vi "Manual Assembly DB new.vi"() -> ()   [LabVIEW 2021]
uses:
  Classes/Routine/Routine Enum.ctl
  Classes/Assembly/Database Entry/Database Entry.lvclass
  Classes/Assembly/Assembly Run.lvclass
  Classes/Workspace/Fixture Enum.ctl
  <vilib>/Utility/file.llb/Read Delimited Spreadsheet (string).vi
  SubVIs/PUT_region.vi
  SubVIs/component_tray_region.vi
  SubVIs/assembly_tray_region.vi
  Classes/Routine/Routine.lvclass
  Classes/Workspace/Fixture.lvclass
  Classes/Controller/Controller.lvclass
  <vilib>/JDP Science/JDP Science Common Utilities/JDP Utility.lvlib
panel:
  out "Stack names":T1
  out "Feet check":bool
  out "Assembly Type":string[](array[string])
  out "Assembly tray region":dbl
  out "Component tray region":dbl
  out "PUT Region":dbl
  in  "Clear All":bool
  in  "Assemble":bool
  in  "Pick and Place":bool
  in  "Dispense glue":bool
  in  "Go":bool
  in  "Routine":T2=enum."Dispense Epoxy"
  in  "Update":bool
  in  "Stage":i32(listbox)=-1
  in  "Stop":bool
  in  "Remove":bool
  in  "Add":bool
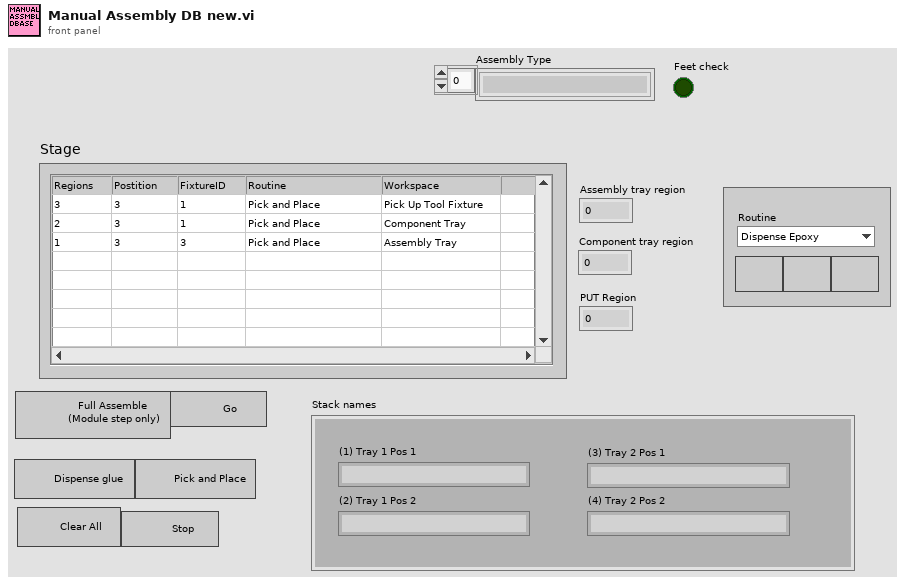
[diagram p1: front panel]
types:
  T1 = cluster{"(1) Tray 1 Pos 1":string, "(2) Tray 1 Pos 2":string, "(3) Tray 2 Pos 1":string, "(4) Tray 2 Pos 2":string}
  T2 = typedef "Routine.lvclass/Routine Enum.ctl" = enum16{"Primary Pick Up", "Secondary Pick Up", "Put Down All", "Secure Syringe", "Release Syringe", "Dispense Epoxy", "Pick Up All", "Put Down Secondary", "Full Assembly"}
  T3 = typedef "Fixture.lvclass/Fixture Enum.ctl" = enum16{"Assembly Tray", "Syringe Space", "Component", "Pick Up Tool", "Current Position"}
  T4 = typedef "File Paths.ctl" = cluster{"Glue Pattern Folder":path, "Carrier Tray Folder":path, "Pick Up Tool Fixture Folder":path, "Components Folder":path, "Bellows Tool Offset.txt":path, "Pick Up Tool Offset.txt":path, "Dispense Tip Offset.txt":path, "Log Files":path, "Gantry Assembly Map.txt":path, "Syringe and offset map.txt":path, "Controllers Folder":path, "Local dbase config":path}
  T5 = cluster{"Fixture ID":dbl, "Position":dbl, "Thickness":dbl}[]
  T6 = cluster{"Stack names[0]":string, "Stack names[1]":string, "Stack names[2]":string, "Stack names[3]":string}
  T7 = typedef "Controller.lvclass/Controllers.ctl" = cluster{"I-O.lvclass":refnum<class "I-O.lvclass">, "Gantry":refnum<k24>, "Dispenser":refnum<visa-resource-name>}
  T8 = cluster{"Fixture ID":dbl, "Position":dbl, "Thickness":dbl}
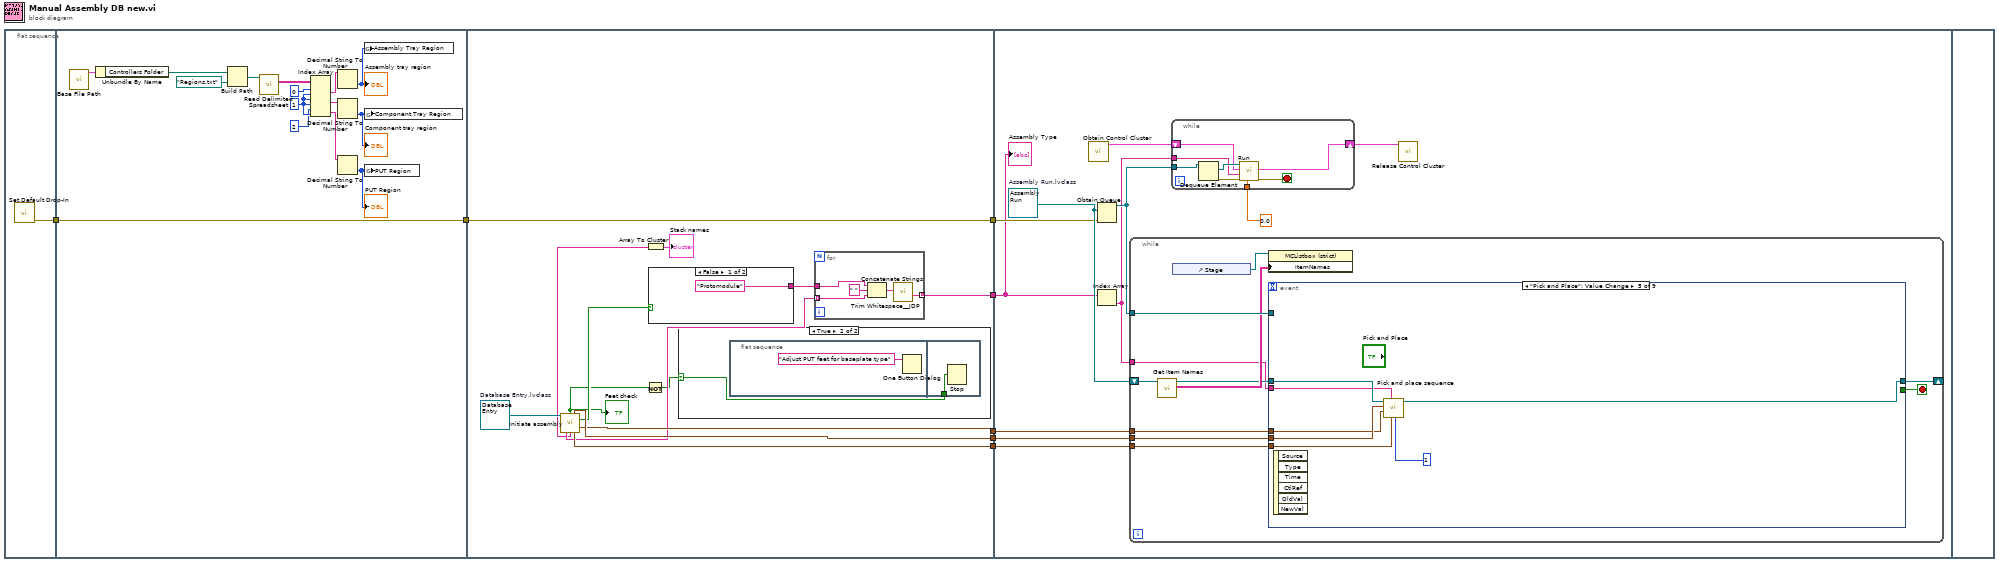
[diagram p0: block diagram]
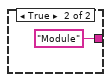
[diagram p3: hidden frame]
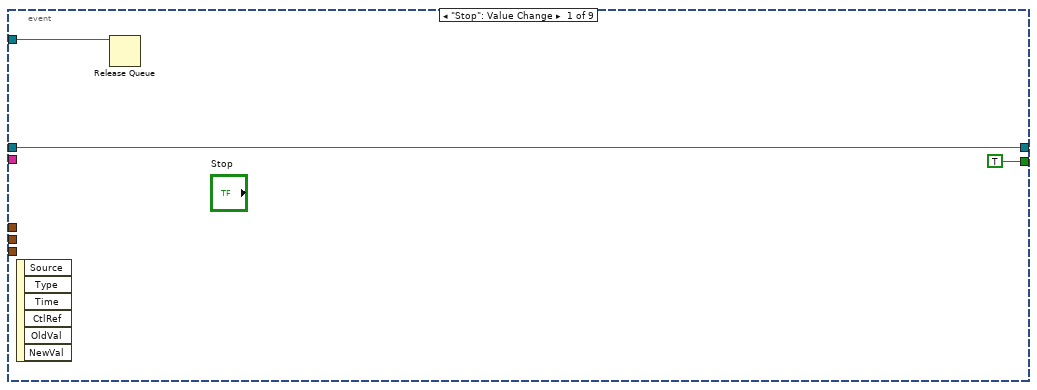
[diagram p4: hidden frame]
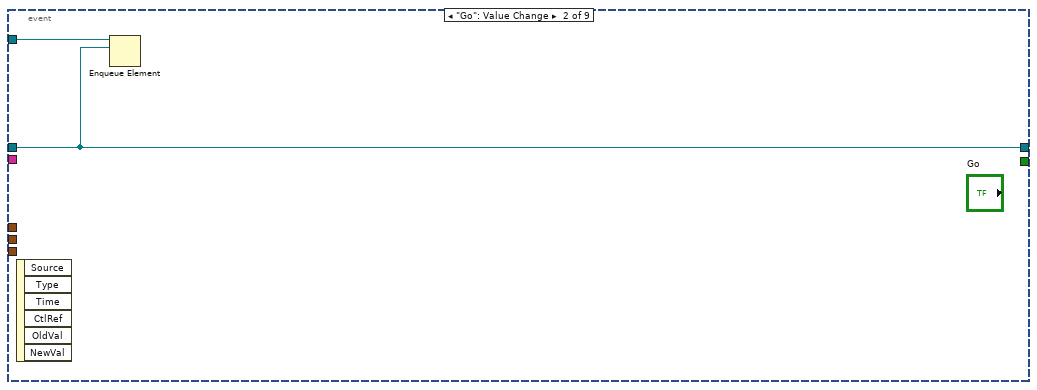
[diagram p5: hidden frame]
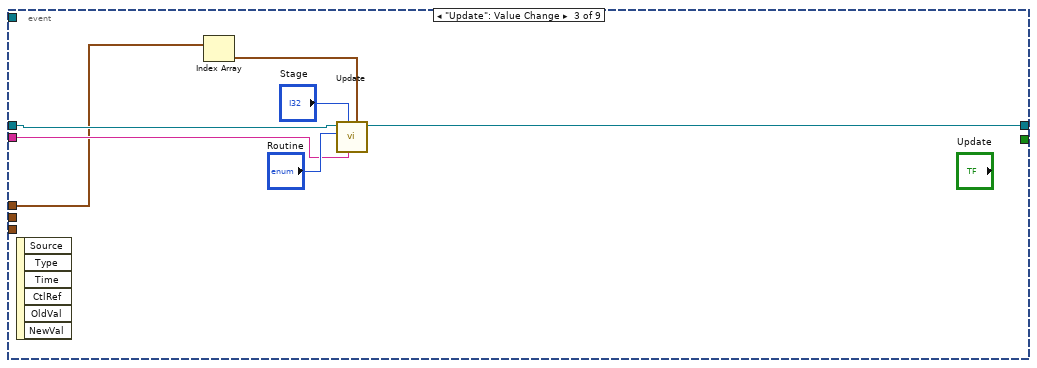
[diagram p6: hidden frame]
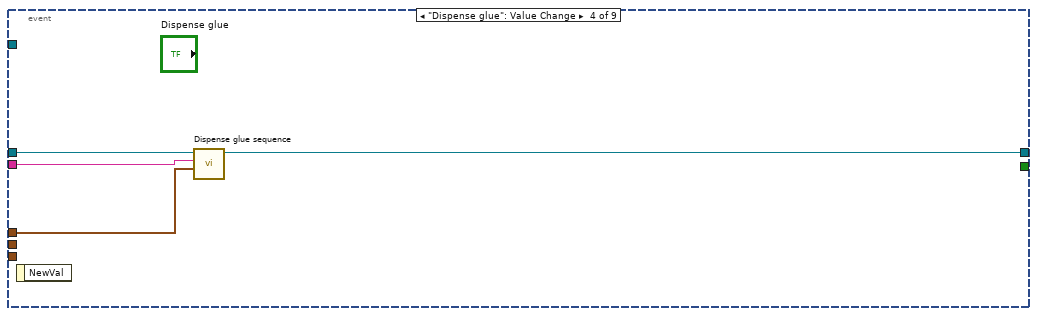
[diagram p7: hidden frame]
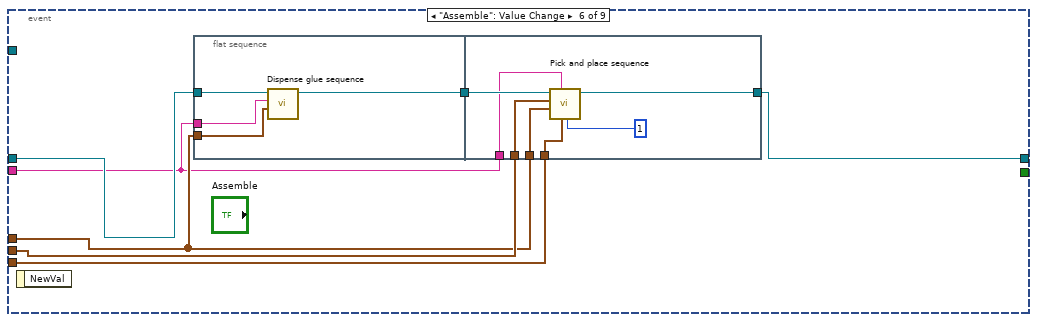
[diagram p8: hidden frame]
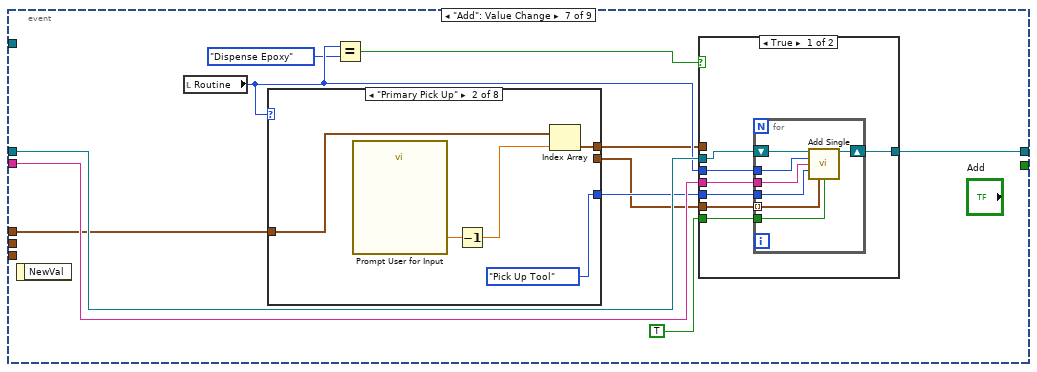
[diagram p9: hidden frame]
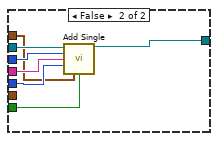
[diagram p10: hidden frame]
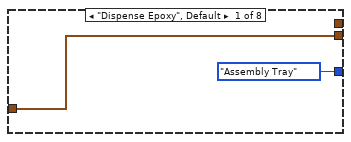
[diagram p11: hidden frame]
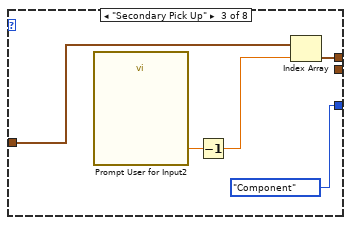
[diagram p12: hidden frame]
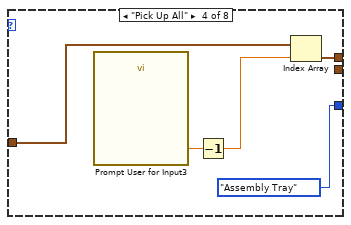
[diagram p13: hidden frame]
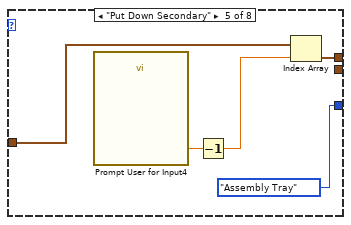
[diagram p14: hidden frame]
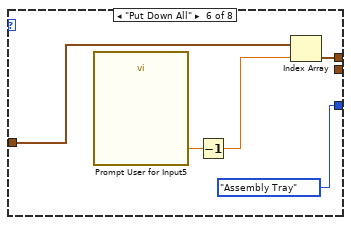
[diagram p15: hidden frame]
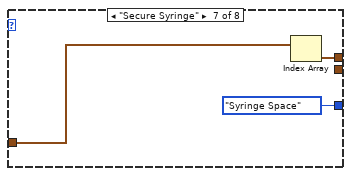
[diagram p16: hidden frame]
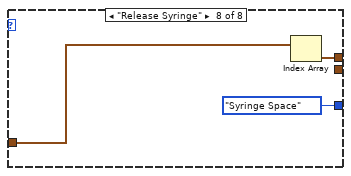
[diagram p17: hidden frame]
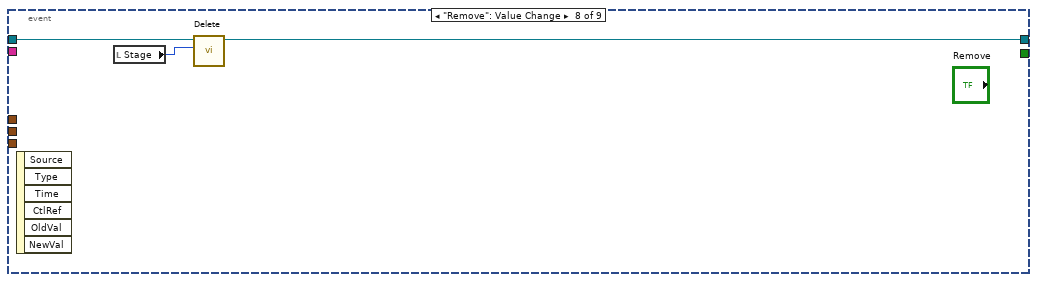
[diagram p18: hidden frame]
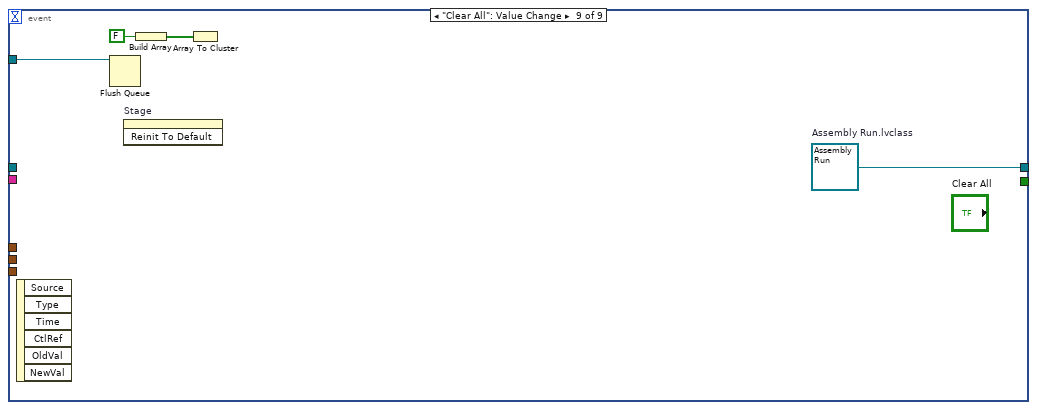
[diagram p19: hidden frame]
diagram:
  n1 = flat-sequence {
    tunnel: [w8] -> w5
    tunnel: [w9] -> w6
    tunnel: w5 -> [w9]
    tunnel: [w35] -> w7
    tunnel: w6 -> [w35]
    tunnel: [w34] -> w4
    tunnel: [w33] -> w3
    tunnel: [w32] -> w2
    tunnel: [w28] -> w1
    tunnel: w7 -> [w53]
    tunnel: w4 -> [w52]
    tunnel: w3 -> [w51]
    tunnel: w2 -> [w50]
    tunnel: w1 -> [w49]
    frame #0 {
      n2 = call "Set Default Drop-In.vi"() -> ("error out"=w8:errorcluster)  [unwired: 11 in]
    }
    frame #1 {
      w12 = 1 ("disabled index (col)")
      n3 = call "Base File Path.vi"() -> ("Paths Out"=w23:T4)  [unwired: 11 in]
      n4 = Unbundle By Name(w23) -> ("Controllers Folder"=w21:path)
      n5 = Build Path(base path=w21, name or relative path=path "Regions.txt") -> (appended path=w22:path)
      n6 = call-poly <vilib>:"Read Delimited Spreadsheet.vi"("file path (dialog if empty)"=w22) -> ("all rows"=w10:string[][])  [unwired: 9 in, 5 out]
      n7 = Index Array(array=w10, index (row) #1=0 ("index (row)"), index (col) #1=w12, index (row) #2=w12, index (col) #2=w12, index (row) #3=2 ("disabled index (row)"), index (col) #3=w12) -> (element #1=w15:string, element #2=w14:string, element #3=w16:string)
      n8 = Decimal String To Number(string=w15) -> (number=w18:i32)  [unwired: 2 in, 1 out]
      "Assembly tray region" <- w18
      n9 = Decimal String To Number(string=w14) -> (number=w19:i32)  [unwired: 2 in, 1 out]
      "Component tray region" <- w19
      n10 = Decimal String To Number(string=w16) -> (number=w17:i32)  [unwired: 2 in, 1 out]
      "PUT Region" <- w17
      n11 = global write "assembly_tray_region.vi" "Assembly Tray Region"(w18) -> ()
      n12 = global write "component_tray_region.vi" "Component Tray Region"(w19) -> ()
      n13 = global write "PUT_region.vi" "PUT Region"(w17) -> ()
    }
    frame #2 {
      w36 = refnum<class "Database Entry.lvclass"> refnum  # Database Entry.lvclass
      n14 = call "Initiate assembly.vi"("Database Entry in"=w36) -> ("Feet check"=w24:bool, "PUT Settings"=w33:T5, "Module?"=w31:bool, "Assembly Settings"=w32:T5, "Assembly Type"=w30:string[], "Stack names"=w25:string[], "Component Settings"=w34:T5)  [unwired: 5 in, 3 out]
      "Feet check" <- w24
      n15 = Array To Cluster(array=w25) -> (cluster=→"Stack names":T6)
      n16 = Not(x=w24) -> (.not. x?=w27:bool)
      n17 = case shown="False" w31 {
        tunnel: ["Protomodule" "Module"] -> w29
        frame False {
        }
        frame True {
        }
      }
      n18 = case shown="True" w27 {
        selector: w27 -> [_ w37]
        frame False {
        }
        frame True {
          n19 = flat-sequence {
            tunnel: w37 -> [w39]
            frame #0 {
              n20 = One Button Dialog(message="Adjust PUT feet for baseplate type") -> ()  [unwired: 1 in, 1 out]
            }
            frame #1 {
              n21 = Stop(stop? (T)=w39) -> ()
            }
          }
        }
      }
      n22 = for {
        tunnel: w30 -> [w42] mode=indexing
        tunnel: w29 -> [w44]
        tunnel: [w40] -> w28 mode=indexing
        n23 = Concatenate Strings(w44, " " ("string"), w42) -> (w41:string)
        n24 = call <vilib>:"Trim Whitespace__JDP.vi"("String in"=w41) -> ("String out"=w40:string)  [unwired: 6 in]
      }
    }
    frame #3 {
      w55 = refnum<class "Assembly Run.lvclass"> refnum  # Assembly Run.lvclass
      n25 = call "Obtain Control Cluster.vi"() -> ("Control Out"=w54:T7)  [unwired: 11 in]
      n26 = Obtain Queue(element data type=w55, error in (no error)=w53) -> (queue out=w57:refnum<queue>)  [unwired: 3 in, 2 out]
      n27 = Index Array(array=w49) -> (element=w48:string)  [unwired: 1 in]
      n28 = while {
        shift-right: [w62] -> _
        shift-left: w55 -> [w64]
        tunnel: w57 -> [w67]
        tunnel: w52 -> [w61]
        tunnel: w51 -> [w60]
        tunnel: w50 -> [w59]
        tunnel: w48 -> [w58]
        stop <- w68 stop-if-true
        n29 = call "Get Item Names.vi"("Assembly Run in"=w64) -> ("Item names"=w66:string[][], "Assembly Run out"=w63:refnum<class "Assembly Run.lvclass">)  [unwired: 8 in, 1 out]
        n30 = control-ref of="Stage"() -> (w65:refnum<vi>)
        n31 = property class="MCListbox (strict)"(reference=w65, "ItemNames"=w66) -> ()  [unwired: 1 in, 2 out]
        n32 = event shown="[4] \"Pick and Place\": Value Change" {
          selector: _ -> [_ _ _ _ _ _ _ _ _]
          dyn-events: _ -> [_ _ _ _ _ _ _ _ _]
          timeout: _ -> [_ _ _ _ _ _ _ _ _]
          tunnel: [TRUE _ _ _ _ _ _ _ _] -> w68
          tunnel: w63 -> [w70 w72 w80 w84 w91 w98 w119 w177 _]
          tunnel: [w70 w72 w79 w83 w90 w97 w120 w176 w181] -> w62
          tunnel: w67 -> [w69 w73 _ _ _ _ _ _ w180]
          tunnel: w61 -> [_ _ _ _ w85 w94 _ _ _]
          tunnel: w60 -> [_ _ _ _ w89 w95 _ _ _]
          tunnel: w59 -> [_ _ w75 w82 w86 w93 w115 _ _]
          tunnel: w58 -> [_ _ w76 w81 w88 w92 w118 _ _]
          event "Stop": Value Change {
            n33 = event-data() -> ()  [unwired: 1 in, 6 out]
            n34 = Release Queue(queue=w69) -> ()  [unwired: 2 in, 3 out]
          }
          event "Go": Value Change {
            n35 = event-data() -> ()  [unwired: 1 in, 6 out]
            n36 = Enqueue Element(queue=w73, element=w72) -> ()  [unwired: 2 in, 3 out]
          }
          event "Update": Value Change {
            n37 = event-data() -> ()  [unwired: 1 in, 6 out]
            n38 = Index Array(array=w75) -> (element=w74:T8)  [unwired: 1 in]
            n39 = call "Update.vi"("Input Settings"=w74, "Assembly Type"=w76, "Row"="Stage", "Routine"="Routine", "Assembly Run in"=w80) -> ("Assembly Run out"=w79:refnum<class "Assembly Run.lvclass">)  [unwired: 5 in, 1 out]
          }
          event "Dispense glue": Value Change {
            n40 = event-data() -> ()  [unwired: 1 in, 1 out]
            n41 = call "Dispense glue sequence.vi"("Assembly Tray Settings Array"=w82, "Assembly Type"=w81, "Assembly Run in"=w84) -> ("Assembly Run out"=w83:refnum<class "Assembly Run.lvclass">)  [unwired: 7 in, 1 out]
          }
          event "Pick and Place": Value Change {
            n42 = event-data() -> ()  [unwired: 1 in, 6 out]
            n43 = call "Pick and place sequence.vi"("Numeric"=1, "Component Tray map"=w85, "Assembly Type"=w88, "Assembly Tray map"=w86, "PUT map"=w89, "Assembly Run in"=w91) -> ("Assembly Run out"=w90:refnum<class "Assembly Run.lvclass">)  [unwired: 4 in, 1 out]
          }
          event "Assemble": Value Change {
            n44 = event-data() -> ()  [unwired: 1 in, 1 out]
            n45 = flat-sequence {
              tunnel: [w101] -> w96
              tunnel: w98 -> [w102]
              tunnel: w93 -> [w100]
              tunnel: w92 -> [w99]
              tunnel: [w108] -> w97
              tunnel: w96 -> [w109]
              tunnel: w93 -> [w107]
              tunnel: w95 -> [w106]
              tunnel: w94 -> [w105]
              tunnel: w92 -> [w104]
              frame #0 {
                n46 = call "Dispense glue sequence.vi"("Assembly Tray Settings Array"=w100, "Assembly Type"=w99, "Assembly Run in"=w102) -> ("Assembly Run out"=w101:refnum<class "Assembly Run.lvclass">)  [unwired: 7 in, 1 out]
              }
              frame #1 {
                n47 = call "Pick and place sequence.vi"("Numeric"=1, "Component Tray map"=w105, "Assembly Type"=w104, "Assembly Tray map"=w107, "PUT map"=w106, "Assembly Run in"=w109) -> ("Assembly Run out"=w108:refnum<class "Assembly Run.lvclass">)  [unwired: 4 in, 1 out]
              }
            }
          }
          event "Add": Value Change {
            n48 = event-data() -> ()  [unwired: 1 in, 1 out]
            n49 = local read "Routine"() -> (w113:T2)
            n50 = case shown="\"Primary Pick Up\"" w113 {
              tunnel: [Fixture_Enum."Assembly Tray" ("Fixture") Fixture_Enum."Pick Up Tool" ("Fixture") Fixture_Enum."Component" ("Fixture") Fixture_Enum."Assembly Tray" ("Fixture") Fixture_Enum."Assembly Tray" ("Fixture") Fixture_Enum."Assembly Tray" ("Fixture") Fixture_Enum."Syringe Space" ("Fixture") Fixture_Enum."Syringe Space" ("Fixture")] -> w117
              tunnel: w115 -> [w142 w147 w150 w155 w160 w164 w170 w173]
              tunnel: [_ w144 w149 w154 w159 w165 w169 w172] -> w110
              tunnel: [w142 _ _ _ _ _ _ _] -> w111
              frame "Dispense Epoxy", Default {
              }
              frame "Primary Pick Up" {
                n51 = call "Prompt User for Input"() -> ("Position"=w146:dbl)  [unwired: 17 in, 2 out]
                n52 = Decrement(x=w146) -> (x-1=w145:dbl)
                n53 = Index Array(array=w147, index=w145) -> (element=w144:T8)
              }
              frame "Secondary Pick Up" {
                n54 = call "Prompt User for Input2"() -> ("Position"=w152:dbl)  [unwired: 17 in, 2 out]
                n55 = Decrement(x=w152) -> (x-1=w151:dbl)
                n56 = Index Array(array=w150, index=w151) -> (element=w149:T8)
              }
              frame "Pick Up All" {
                n57 = call "Prompt User for Input3"() -> ("Position"=w157:dbl)  [unwired: 17 in, 2 out]
                n58 = Decrement(x=w157) -> (x-1=w156:dbl)
                n59 = Index Array(array=w155, index=w156) -> (element=w154:T8)
              }
              frame "Put Down Secondary" {
                n60 = call "Prompt User for Input4"() -> ("Position"=w162:dbl)  [unwired: 17 in, 2 out]
                n61 = Decrement(x=w162) -> (x-1=w161:dbl)
                n62 = Index Array(array=w160, index=w161) -> (element=w159:T8)
              }
              frame "Put Down All" {
                n63 = call "Prompt User for Input5"() -> ("Position"=w167:dbl)  [unwired: 17 in, 2 out]
                n64 = Decrement(x=w167) -> (x-1=w166:dbl)
                n65 = Index Array(array=w164, index=w166) -> (element=w165:T8)
              }
              frame "Secure Syringe" {
                n66 = Index Array(array=w170) -> (element=w169:T8)  [unwired: 1 in]
              }
              frame "Release Syringe" {
                n67 = Index Array(array=w173) -> (element=w172:T8)  [unwired: 1 in]
              }
            }
            n68 = Equal?(x=w113, y=Routine_Enum."Dispense Epoxy") -> (x = y?=w114:bool)
            n69 = case shown="True" w114 {
              tunnel: [w127 w141] -> w120
              tunnel: w119 -> [w126 w140]
              tunnel: w118 -> [w125 w139]
              tunnel: w117 -> [w124 w138]
              tunnel: w113 -> [w123 w137]
              tunnel: TRUE ("Auto") -> [w122 w136]
              tunnel: w111 -> [w121 _]
              tunnel: w110 -> [_ w135]
              frame True {
                n70 = for {
                  tunnel: w125 -> [w132]
                  tunnel: w124 -> [w131]
                  tunnel: w123 -> [w130]
                  tunnel: w122 -> [w129]
                  shift-right: [w134] -> w127
                  shift-left: w126 -> [w133]
                  tunnel: w121 -> [w128] mode=indexing
                  n71 = call-dynamic "Add Single.vi"("UI in"=w133, "Routine"=w130, "Assembly Type"=w132, "Fixture"=w131, "Input Settings"=w128, "Auto"=w129) -> ("UI out"=w134:refnum<class "Assembly Run.lvclass">)  [unwired: 8 in, 1 out]
                }
              }
              frame False {
                n72 = call-dynamic "Add Single.vi"("UI in"=w140, "Routine"=w137, "Assembly Type"=w139, "Fixture"=w138, "Input Settings"=w135, "Auto"=w136) -> ("UI out"=w141:refnum<class "Assembly Run.lvclass">)  [unwired: 8 in, 1 out]
              }
            }
          }
          event "Remove": Value Change {
            n73 = event-data() -> ()  [unwired: 1 in, 6 out]
            n74 = local read "Stage"() -> (w175:i32)
            n75 = call "Delete.vi"("Index"=w175, "Assembly In"=w177) -> ("Assembly Out"=w176:refnum<class "Assembly Run.lvclass">)  [unwired: 8 in, 1 out]
          }
          event "Clear All": Value Change {
            w181 = refnum<class "Assembly Run.lvclass"> refnum  # Assembly Run.lvclass
            n76 = event-data() -> ()  [unwired: 1 in, 6 out]
            n77 = Flush Queue(queue=w180) -> ()  [unwired: 1 in, 3 out]
            n78 = invoke on="Stage" class="MCListbox (strict)" method="Reinit To Default"() -> ()  [unwired: 3 in, 3 out]
            n79 = Build Array(FALSE) -> (w179:bool[])
            n80 = Array To Cluster(array=w179) -> ()  [unwired: 1 out]
          }
        }
      }
      n81 = while {
        tunnel: w57 -> [w189]
        shift-right: [w184] -> w56
        shift-left: w54 -> [w185]
        tunnel: w48 -> [w183]
        tunnel: 0.0 -> [w182]
        stop <- w186 stop-if-true
        n82 = Dequeue Element(queue=w189) -> (element=w188:refnum<class "Assembly Run.lvclass">, error out=w187:errorcluster)  [unwired: 2 in, 2 out]
        n83 = call-dynamic "Run.vi"("Pickup_Test_Number"=w182, "error in (no error)"=w187, "Assembly Type"=w183, "Control In"=w185, "Assembly In"=w188) -> ("error out"=w186:errorcluster, "Control Out"=w184:T7)  [unwired: 4 in, 1 out]
      }
      n84 = call "Release Control Cluster.vi"("output cluster"=w56) -> ()  [unwired: 11 in]
      "Assembly Type" <- w49
    }
    frame #4 {
    }
  }
